vi "ep_Generate Pulse Signal.vi"(0 "trigger signal? (F)":bool, 7 "pulse duration [ms]":u32) -> (4 "pulse signal?":bool)   [LabVIEW 2012]
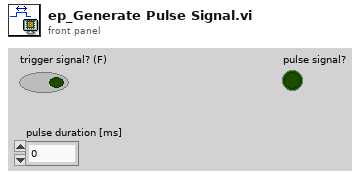
[diagram p1: front panel]
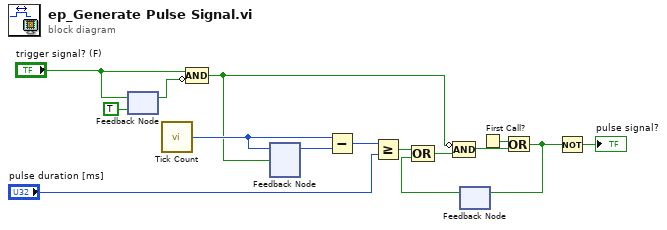
[diagram p0: block diagram]
diagram:
  n1 = feedback #1(TRUE ("trigger signal? (F)")) -> (w4:bool)
  n2 = feedback-in #1("trigger signal? (F)") -> ()
  n3 = call "Tick Count"() -> ("Tick Count(mSec)"=w11:u32)
  n4 = Compound Arithmetic op=AND("trigger signal? (F)", invert w4) -> (w2:bool)
  n5 = feedback #2() -> (w15:u32)  [unwired: 1 in]
  n6 = feedback-in #2(w11, w2) -> ()
  n7 = Subtract(x=w11, y=w15) -> (x-y=w14:u32)
  n8 = Greater Or Equal?(x=w14, y="pulse duration [ms]") -> (x >= y?=w7:bool)
  n9 = feedback #3() -> (w6:bool)  [unwired: 1 in]
  n10 = Compound Arithmetic op=OR(w7, w6) -> (w12:bool)
  n11 = Compound Arithmetic op=AND(invert w2, w12) -> (w9:bool)
  n12 = First Call?() -> (First Call?: T/F=w10:bool)
  n13 = Or(x=w10, y=w9) -> (x .or. y?=w8:bool)
  n14 = feedback-in #3(w8) -> ()
  n15 = Not(x=w8) -> (.not. x?=→"pulse signal?":bool)
